vi "Read Numeric Control.vi"(8 "error in (no error)":errorcluster, 11 "ParentClass in":refnum<class "ParentClass.lvclass">) -> (0 "error out":errorcluster, 2 "Numeric Control":dbl, 3 "ParentClass out":refnum<class "ParentClass.lvclass">)   [LabVIEW 2012, in "ParentClass.lvclass"]
uses:
  ParentClass.lvclass
  ParentClass.lvclass/ParentClass.ctl
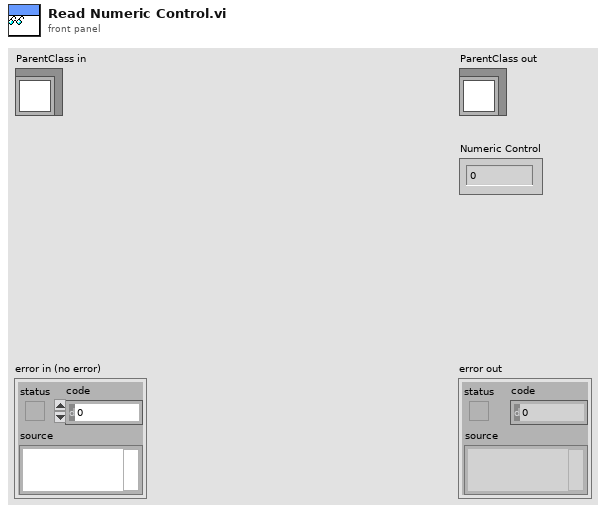
[diagram p1: front panel]
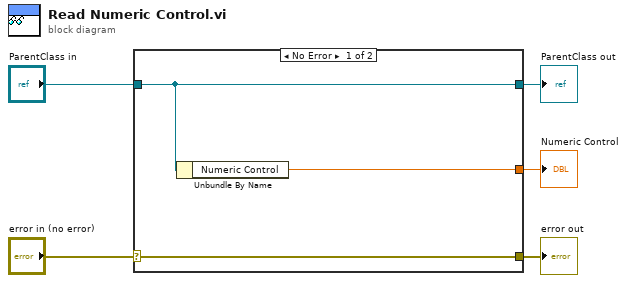
[diagram p0: block diagram]
diagram:
  n1 = case shown="No Error" "error in (no error)" {
    selector: "error in (no error)" -> [w8 w9]
    tunnel: [w8 w9] -> w4
    tunnel: [w7 w10] -> w2
    tunnel: "ParentClass in" -> [w7 w10]
    tunnel: [w6 _] -> w1
    frame No Error {
      n2 = Unbundle By Name(w7) -> ("Numeric Control"=w6:dbl)
    }
    frame Error {
    }
  }
  "error out" <- w4
  "ParentClass out" <- w2
  "Numeric Control" <- w1
